vi "DestroyPrivateEvents.vi"(8 "error in (no error)":errorcluster, 11 "XYStage.KIM101":refnum<class "XYStage.KIM101.lvclass">) -> (0 "error out":errorcluster, 3 "XYStage.KIM101 out":refnum<class "XYStage.KIM101.lvclass">)   [LabVIEW 2017, in "XYStage.KIM101.lvclass"]
doc: "JKI State Machine Objects (SMO) 1.3.0.56\nJKI - JKI\nCopyright (c) 2017, JKI"
uses:
  XYStage.KIM101.lvclass
  XYStage/XYStage.lvclass
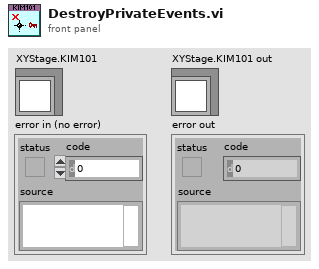
[diagram p1: front panel]
types:
  T1 = typedef "XYStage.KIM101.lvclass/PrivateEvents--Cluster.ctl" = cluster{"MoveAbsolute (counts)":refnum<user-event>}
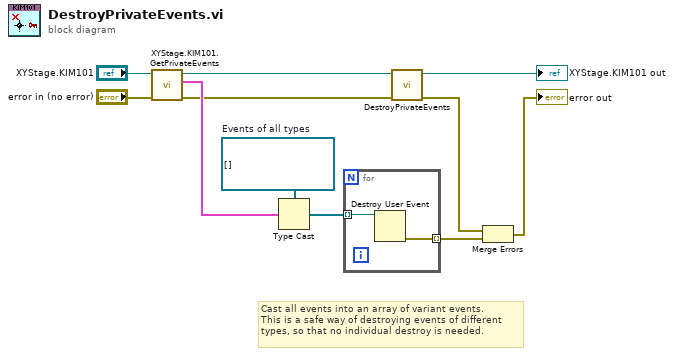
[diagram p0: block diagram]
diagram:
  w9 = refnum<user-event>[] []  # Events of all types
  # "Cast all events into an array of variant events.\nThis is a safe way of destroying events of different\ntypes, so that no individual destroy is needed."
  n1 = call "XYStage.KIM101.GetPrivateEvents.vi"("error in (no error)"="error in (no error)", "XYStage.KIM101 in"="XYStage.KIM101") -> ("error out"=w4:errorcluster, "Private Events"=w6:T1, "XYStage.KIM101 out"=w5:refnum<class "XYStage.KIM101.lvclass">)  [unwired: 7 in]
  n2 = Type Cast(type=w9, x=w6) -> (*(type *) &x=w8:refnum<user-event>[])
  n3 = for {
    tunnel: w8 -> [w13] mode=indexing
    tunnel: [w12] -> w7 mode=indexing
    n4 = Destroy User Event(user event=w13) -> (error out=w12:errorcluster)  [unwired: 1 in]
  }
  n5 = call-parent "DestroyPrivateEvents.vi"("error in (no error)"=w4, "XYStage"=w5) -> ("error out"=w3:errorcluster, "XYStage out"=→"XYStage.KIM101 out":refnum<class "XYStage.KIM101.lvclass">)  [unwired: 8 in]
  n6 = Merge Errors(w3, w7) -> (→"error out":errorcluster)
